vi "Counter.vi"(9 "step":u32=1, 10 "enable":bool=TRUE, 11 "limit":u32) -> (2 "count = limit?":bool, 3 "count":u32)   [LabVIEW 2017]
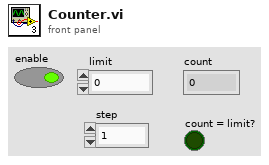
[diagram p1: front panel]
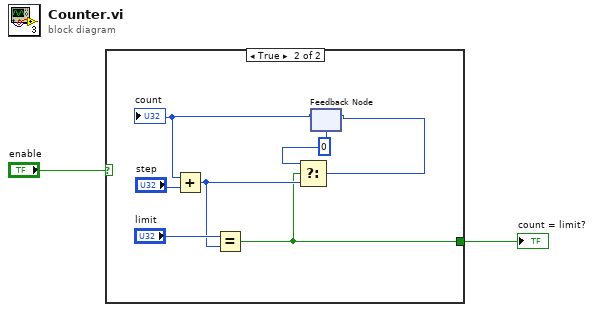
[diagram p0: block diagram]
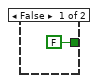
[diagram p2: hidden frame]
diagram:
  n1 = case shown="True" "enable" {
    tunnel: [FALSE w4] -> w1
    frame False {
    }
    frame True {
      w10 = u32 0
      n2 = feedback #1(w10) -> (w6:u32)
      "count" <- w6
      n3 = Add(x=w6, y="step") -> (x+y=w5:u32)
      n4 = Equal?(x="limit", y=w5) -> (x = y?=w4:bool)
      n5 = Select(t=w10, s=w4, f=w5) -> (s? t:f=w8:u32)
      n6 = feedback-in #1(w8) -> ()
    }
  }
  "count = limit?" <- w1
